vi "Update Values.vi"(8 "error in":errorcluster, 11 "Robot Mode":T1) -> (0 "error out":errorcluster)   [LabVIEW 2016]
uses:
  <vilib>/Rock Robotics/WPI/DriverStation/WPI_DriverStationRobotMode2.ctl
  2017 Robot Project/Framework/Robot Global Data.vi
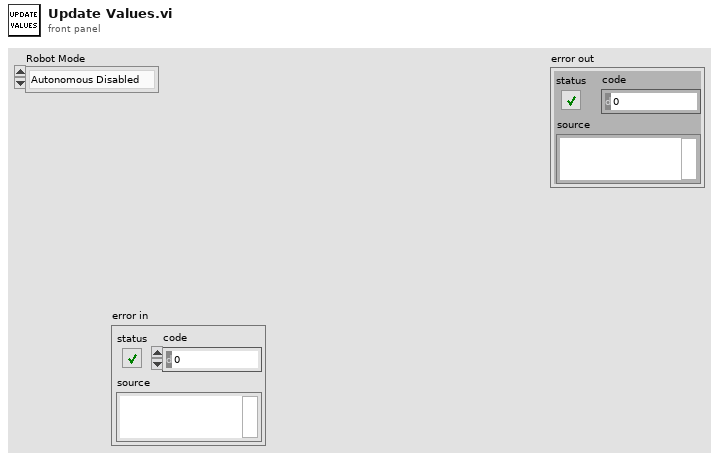
[diagram p1: front panel]
types:
  T1 = typedef "WPI_DriverStationRobotMode2.ctl" = enum16{"Autonomous Disabled", "Autonomous Enabled", "Teleop Disabled", "Teleop Enabled", "Disconnected", "Finish", "Test Disabled", "Test Enabled", "Emergency Stopped"}
  T2 = typedef "PID Settings.ctl" = cluster{"D":dbl, "F":dbl, "RR":dbl, "IZ":dbl, "P":dbl, "I":dbl}
  T3 = typedef "NI_LVConfig.lvlib/Config Data RefNum.ctl" = refnum<k1>
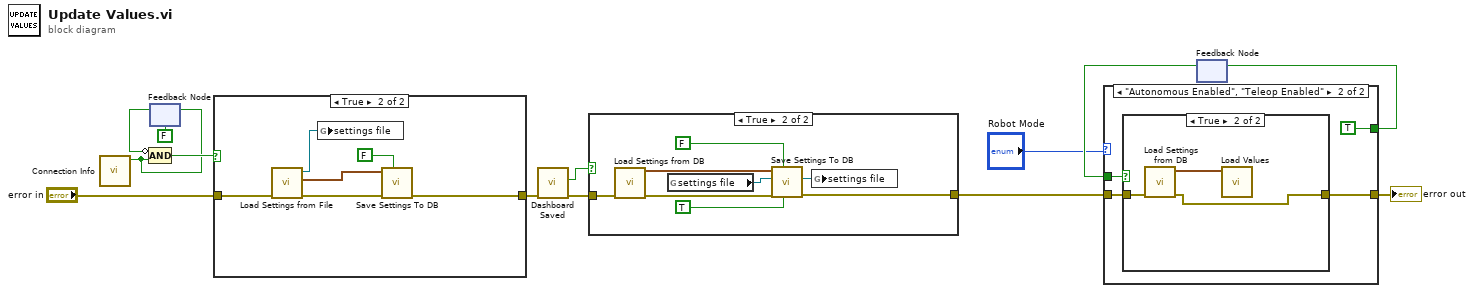
[diagram p0: block diagram]
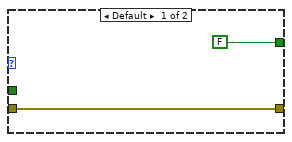
[diagram p3: hidden frame]
diagram:
  n1 = call <vilib>:"Connection Info.vi"() -> ("Connected"=w1:bool)  [unwired: 10 in, 1 out]
  n2 = feedback-in #1(w1) -> ()
  n3 = feedback #1(FALSE) -> (w4:bool)
  n4 = Compound Arithmetic op=AND(invert w4, w1) -> (w2:bool)
  n5 = case shown="True" w2 {
    tunnel: [w14 w16] -> w6
    tunnel: "error in" -> [w14 w15]
    frame False {
    }
    frame True {
      n6 = call "Load Settings from File.vi"("error in"=w15) -> ("error out"=w20:errorcluster, "Drive PID"=w19:T2, "refnum out"=w17:T3)  [unwired: 8 in]
      n7 = global write "Robot Global Data.vi" "settings file"(w17) -> ()
      n8 = call "Save Settings To DB.vi"("Dashboard?"=FALSE, "error in"=w20, "Drive PID"=w19) -> ("error out"=w16:errorcluster)  [unwired: 7 in, 1 out]
    }
  }
  n9 = call "Dashboard Saved.vi"("error in"=w6) -> ("error out"=w13:errorcluster, "RB SAVED?"=w12:bool)  [unwired: 9 in]
  n10 = case shown="True" w12 {
    tunnel: w13 -> [w21 w29]
    tunnel: [w21 w26] -> w11
    frame False {
    }
    frame True {
      n11 = call "Load Settings from DB.vi"("error in"=w29) -> ("error out"=w28:errorcluster, "Drive PID"=w27:T2)  [unwired: 9 in]
      n12 = global read "Robot Global Data.vi" "settings file"() -> (w23:T3)
      n13 = call "Save Settings To DB.vi"("Save To File?"=TRUE, "Dashboard?"=FALSE, "error in"=w28, "save file (in)"=w23, "Drive PID"=w27) -> ("error out"=w26:errorcluster, "save file (out)"=w22:T3)  [unwired: 5 in]
      n14 = global write "Robot Global Data.vi" "settings file"(w22) -> ()
    }
  }
  n15 = feedback #2() -> (w9:bool)  [unwired: 1 in]
  n16 = case shown="\"Autonomous Enabled\", \"Teleop Enabled\"" "Robot Mode" {
    tunnel: w11 -> [w30 w33]
    tunnel: [FALSE TRUE] -> w10
    tunnel: w9 -> [_ w34]
    tunnel: [w30 w32] -> w8
    frame Default {
    }
    frame "Autonomous Enabled", "Teleop Enabled" {
      n17 = case shown="True" w34 {
        tunnel: w33 -> [w36 w39]
        tunnel: [w36 w37] -> w32
        frame False {
        }
        frame True {
          n18 = call "Load Settings from DB.vi"("error in"=w39) -> ("error out"=w37:errorcluster, "Drive PID"=w38:T2)  [unwired: 9 in]
          n19 = call "Load Values.vi"("Drive PID"=w38) -> ()  [unwired: 11 in]
        }
      }
    }
  }
  "error out" <- w8
  n20 = feedback-in #2(w10) -> ()
